vi "Increment Decrement Indent.vi"(8 "error in (no error)":errorcluster, 10 "Increment":bool, 11 "JSON Serializer in":refnum<class "JSON Serializer.lvclass">) -> (0 "error out":errorcluster, 3 "JSON Serializer out":refnum<class "JSON Serializer.lvclass">)   [LabVIEW 2013, in "JKI JSON Serialization.lvlib" / "JSON Serializer.lvclass"]
uses:
  JSON Serializer.lvclass
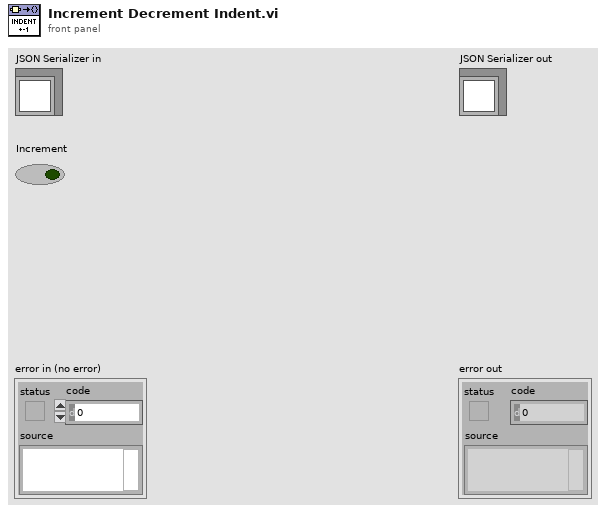
[diagram p1: front panel]
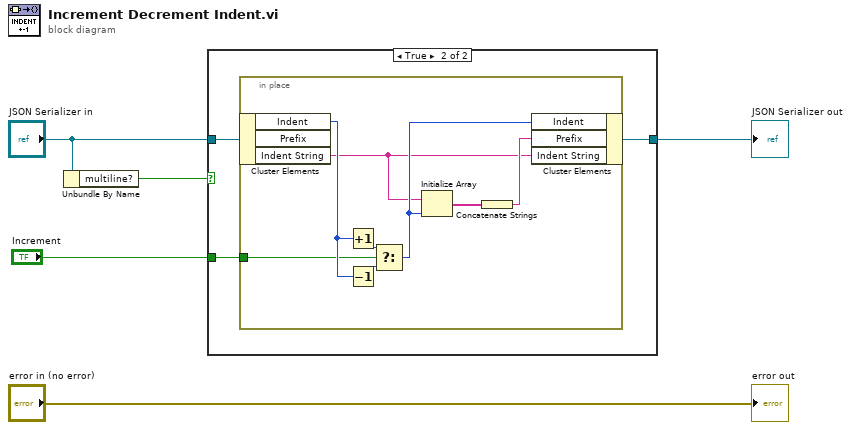
[diagram p0: block diagram]
diagram:
  n1 = Unbundle By Name("JSON Serializer in") -> ("multiline?"=w3:bool)
  n2 = case shown="True" w3 {
    tunnel: [w6 w8] -> w5
    tunnel: "JSON Serializer in" -> [w6 w9]
    tunnel: "Increment" -> [_ w7]
    frame False {
    }
    frame True {
      n3 = in-place {
        in-place-border: w7 -> [w11]
        n4 = in-place-cluster #1(w9) -> ("Indent"=w15:i32, "Indent String"=w10:string)  [unwired: 1 out]
        n5 = Increment(x=w15) -> (x+1=w14:i32)
        n6 = Decrement(x=w15) -> (x-1=w13:i32)
        n7 = Select(t=w14, s=w11, f=w13) -> (s? t:f=w12:i32)
        n8 = Initialize Array(w10, w12) -> (w17:string[])
        n9 = Concatenate Strings(w17) -> (w16:string)
        n10 = in-place-cluster #1("Indent"=w12, "Prefix"=w16, "Indent String"=w10) -> (w8:refnum<class "JSON Serializer.lvclass">)
      }
    }
  }
  "JSON Serializer out" <- w5
  "error out" <- "error in (no error)"
